vi "TryParrySee.vi"(4 "User Parameter":cluster{refnum<vi>, refnum<vi>}, 6 "Control Ref":refnum<k24>, 7 "Event Common Data":T1) -> ()   [LabVIEW 2018]
uses:
  D:/NI LabVIEW/PowerControlWithAT2/REMOTE_SEE_CONTROLLER/RemoteSeeAbleService.dll
  RemoteSeeAbleService.dll
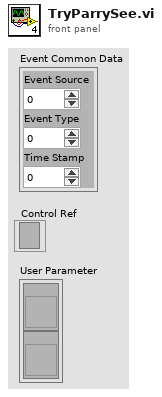
[diagram p1: front panel]
types:
  T1 = cluster{"Event Source":i32, "Event Type":u32, "Time Stamp":u32}
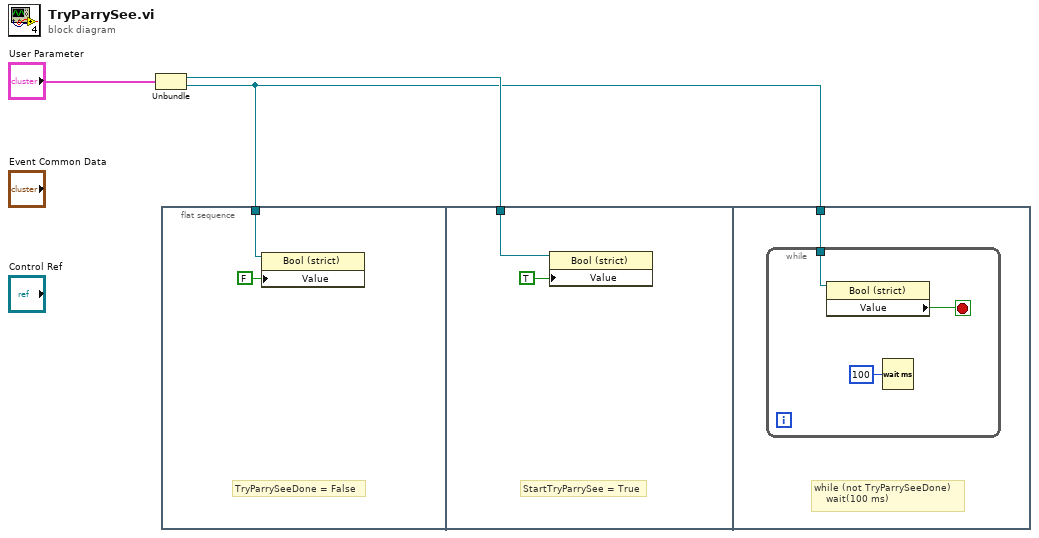
[diagram p0: block diagram]
diagram:
  n1 = Unbundle("User Parameter") -> (w3:refnum<vi>, w2:refnum<vi>)
  n2 = flat-sequence {
    tunnel: w2 -> [w4]
    tunnel: w3 -> [w6]
    tunnel: w2 -> [w8]
    frame #0 {
      # "TryParrySeeDone = False"
      n3 = property class="Bool (strict)"(reference=w4, "Value"=FALSE) -> ()  [unwired: 1 in, 2 out]
    }
    frame #1 {
      # "StartTryParrySee = True"
      n4 = property class="Bool (strict)"(reference=w6, "Value"=TRUE) -> ()  [unwired: 1 in, 2 out]
    }
    frame #2 {
      # "while (not TryParrySeeDone)\n    wait(100 ms)"
      n5 = while {
        tunnel: w8 -> [w9]
        stop <- w11 stop-if-true
        n6 = property class="Bool (strict)"(reference=w9) -> ("Value"=w11:bool)  [unwired: 1 in, 2 out]
        n7 = Wait (ms)(milliseconds to wait=u32 100) -> ()  [unwired: 1 out]
      }
    }
  }
